vi "Insert Sink by Name.vi"(8 "error in (no error)":errorcluster, 9 "Log Sink":refnum<data-value>, 10 "Sink Name":string, 11 "Sink Look Up Table in":refnum<class "Sink Look Up Table.lvclass">) -> (0 "error out":errorcluster, 2 "Replaced?":bool, 3 "Sink Look Up Table out":refnum<class "Sink Look Up Table.lvclass">)   [LabVIEW 2016, in "Stream Log.lvlib" / "Sink Look Up Table.lvclass"]
doc: "--\nCopyright © 2017 Composed SystemsI All rights reserved.\n\nAuthor: Jon McBee <jon.mcbee@composed.io>\n\nThis library is provided \"AS IS\" ,WITHOUT WARRANTIES OR\nCONDITIONS OF ANY KIND, either express or implied.\n\nComposed Systems -- composed.io\n\nStream 0.0.1.1\nJon McBee - Composed Systems\nCopyright (c) 2017, Composed Systems"
uses:
  <userlib>/Composed Systems/Stream/Log/Sink Look Up Table/Sink Look Up Table.lvclass
  C:/Program Files (x86)/National Instruments/LabVIEW 2016/user.lib/Composed Systems/Stream/Look Up Table/Look Up Table/Look Up Table.lvclass
  <userlib>/Composed Systems/Stream/Log/Log Sink/Log Sink.lvclass
  <userlib>/Composed Systems/Stream/Look Up Table/Look Up Table/Look Up Table.lvclass
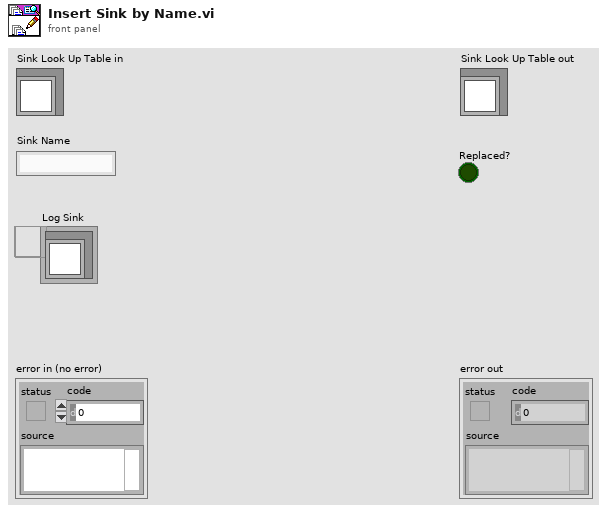
[diagram p1: front panel]
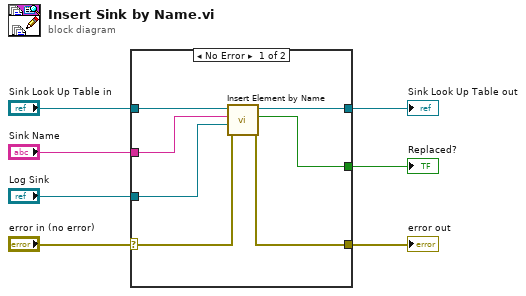
[diagram p0: block diagram]
diagram:
  n1 = case shown="No Error" "error in (no error)" {
    selector: "error in (no error)" -> [w10 w16]
    tunnel: [w9 w16] -> w6
    tunnel: [w13 w15] -> w4
    tunnel: "Sink Look Up Table in" -> [w14 w15]
    tunnel: "Sink Name" -> [w12 _]
    tunnel: "Log Sink" -> [w11 _]
    tunnel: [w8 _] -> w1
    frame No Error {
      n2 = call <userlib>:"Insert Element by Name.vi"("error in (no error)"=w10, "Variant"=w11, "Name"=w12, "Look Up Table in"=w14) -> ("error out"=w9:errorcluster, "Replaced?"=w8:bool, "Look Up Table out"=w13:refnum<class "Sink Look Up Table.lvclass">)  [unwired: 5 in]
    }
    frame Error {
    }
  }
  "error out" <- w6
  "Sink Look Up Table out" <- w4
  "Replaced?" <- w1
